vi "Read Aout Limit Error.vi"(8 "error in (no error)":errorcluster, 11 "VISA resource name":refnum<visa-resource-name>) -> (0 "error out":errorcluster, 2 "aout limit error":cluster{"ALimErrC":bool, "ALimErrL":bool}, 3 "VISA resource name out":refnum<visa-resource-name>)   [LabVIEW 2024, in "Andeen-Hagerling 2700A.lvlib"]
doc: "The analog outputs levels for the capacitance and loss channels\nmay not exceed the upper and lower voltage protection\nlimits. This VI is used to return the status of error reporting\nassociated with this voltage clipping capability."
uses:
  Andeen-Hagerling 2700A.lvlib
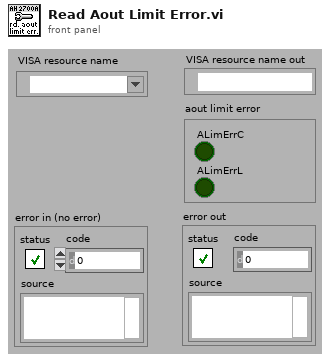
[diagram p1: front panel]
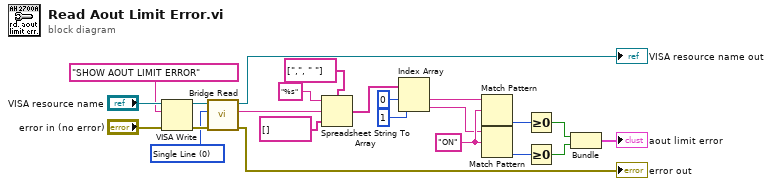
[diagram p0: block diagram]
diagram:
  w1 = u16 0 items=["Single Line", "Multi-Line"] ("Multiline")
  w10 = "ON" ("regular expression")
  n1 = VISA Write(VISA resource name="VISA resource name", write buffer="SHOW AOUT LIMIT ERROR" ("command"), error in (no error)="error in (no error)") -> (VISA resource name out=w21:refnum<visa-resource-name>, error out=w20:errorcluster)  [unwired: 1 out]
  n2 = call "Bridge Read.vi"("error in (no error)"=w20, "multiline"=w1, "VISA resource name"=w21) -> ("error out"=→"error out":errorcluster, "read buffer"=w15:string, "VISA resource name out"=→"VISA resource name out":refnum<visa-resource-name>)  [unwired: 6 in]
  n3 = Spreadsheet String To Array(delimiter (Tab)=string[] [",", " "], format string="%s", spreadsheet string=w15, array type (2D Dbl)=string[] []) -> (array=w11:string[])
  n4 = Index Array(array=w11, index #1=0 ("index"), index #2=1 ("index")) -> (element #1=w9:string, element #2=w8:string)
  n5 = Match Pattern(string=w9, regular expression=w10) -> (offset past match=w7:i32)  [unwired: 1 in, 3 out]
  n6 = Match Pattern(string=w8, regular expression=w10) -> (offset past match=w6:i32)  [unwired: 1 in, 3 out]
  n7 = Greater Or Equal To 0?(x=w7) -> (x >= 0?=w5:bool)
  n8 = Greater Or Equal To 0?(x=w6) -> (x >= 0?=w4:bool)
  n9 = Bundle(w5, w4) -> (→"aout limit error":cluster{bool, bool})  [unwired: 1 in]
